vi "_OLS_Main_Rev2.vi"() -> ()   [LabVIEW 2024]
uses:
  Control Definitions/Def Results2.ctl
  Control Definitions/Def PumpCtlRefs.ctl
  Control Definitions/Def_PumpSpeed.ctl
  Control Definitions/Def TestState.ctl
  Control Definitions/Global 1.vi
  Control Definitions/Global 2.vi
panel:
  out "Index Out":i32
  out "TEST State Out":T1
  in  "Pump Speed":T2=enum."SLOW"
  in  "Num Chan":i32=2
  in  "VISA Refnum in":refnum<visa-resource-name>="COM3"
  out "PumpCtlRef out":T3
  in  "SimPV":bool
  out "Ch B  Sim":dbl
  out "Ch A  Sim":dbl
  out "Root Path":path=path "C:/Users/ff107/OneDrive/Documents/GitHub/PWC-OLS"
  out "File Name":string
  out "Time(ms)":dbl=221.000000000016
  in  "Tank Cal Table":T4={"LSe"=8.5, "LKe"=4.0782, "LMe"=5.542, "LKf"=7.004, "LMf"=2.619, "LSf"=2.0}
  out "Level":bool=TRUE
  out "DataQ":bool=TRUE
  in  "ChA":dbl(slide)=24.489795918367346 scale=0.0..1200.0
  in  "ChB":dbl(slide)=36.73469387755102 scale=0.0..1200.0
  in  "ChB +100":bool
  in  "ChA +100":bool
  in  "Check":bool
  out "Laser (raw)":dbl=5.418700218200684
  out "Results out":T5=[[{"Fill"=0.0, "Drain"=0.0, "Status"=1, "Resistor"=100.77651728439153}, {"Fill"=0.0, "Drain"=0.0, "Status"=1, "Resistor"=100.51009270770467}], [{"Fill"=7.4414529208790405, "Drain"=0.0, "Status"=10, "Resistor"=199.9225077433029}, {"Fill"=7.238431105656106, "Drain"=0.0, "Status"=5, "Resistor"=199.90723695805426}], [{"Fill"=7.01332844493592, "Drain"=0.0, "Status"=5, "Resistor"=299.5771992355265}, {"Fill"=6.753456462357763, "Drain"=0.0, "Status"=10, "Resistor"=299.405945542382}], [{"Fill"=6.5453388658426634, "Drain"=0.0, "Status"=10, "Resistor"=398.9472825404134}, {"Fill"=6.2984555038112795, "Drain"=0.0, "Status"=10, "Resistor"=398.8781708461997}], [{"Fill"=6.077648954516121, "Drain"=0.0, "Status"=10, "Resistor"=498.9171881446158}, {"Fill"=5.838658669949018, "Drain"=0.0, "Status"=10, "Resistor"=498.9668209325864}], [{"Fill"=5.635836474430779, "Drain"=0.0, "Status"=10, "Resistor"=599.1164295543886}, {"Fill"=5.372367525813369, "Drain"=0.0, "Status"=10, "Resistor"=599.0753796448585}], [{"Fill"=5.159054576363429, "Drain"=0.0, "Status"=10, "Resistor"=699.4116005363627}, {"Fill"=4.928457133151359, "Drain"=0.0, "Status"=10, "Resistor"=699.1833846499306}], [{"Fill"=4.711946933490899, "Drain"=0.0, "Status"=10, "Resistor"=799.7085090018842}, {"Fill"=4.472056930994641, "Drain"=0.0, "Status"=10, "Resistor"=799.8411539311372}], [{"Fill"=0.0, "Drain"=0.0, "Status"=2, "Resistor"=0.0}, {"Fill"=0.0, "Drain"=0.0, "Status"=0, "Resistor"=0.0}], [{"Fill"=0.0, "Drain"=0.0, "Status"=0, "Resistor"=0.0}, {"Fill"=0.0, "Drain"=0.0, "Status"=0, "Resistor"=0.0}], [{"Fill"=0.0, "Drain"=0.0, "Status"=0, "Resistor"=0.0}, {"Fill"=0.0, "Drain"=0.0, "Status"=0, "Resistor"=0.0}]] {"Resistor" format="%.1f"; "Drain" format="%.3f"; "Fill" format="%.3f"}
  in  "DUT":i16=1
  in  "Pump JOG":bool
  in  "Run Test":bool
  in  "Normal":cluster{u32, u32}[](array[cluster])=[{16711680, 1244948}]
  in  "Sim Color":cluster{u32, u32}[](array[cluster])=[{16774656, 1244948}]
  out "Level \nStatus":bool=TRUE
  out "DataQ\nStatus":bool=TRUE
  in  "Level SP":dbl(slide)=2.6 scale=8.5..2.0
  in  "Level PV":dbl(slide)=4.203692297209104 scale=8.5..2.0
  out "Level":dbl=4.203692297209104 format="%.3f"
  in  "Drain":bool
  in  "Fill":bool
  in  "Simulate":bool
  out "TEST NME":string="OLR001--Junk"
  out "DataQ Input":T6(graph)={"ChA Ohms"=799.7643554010987, "ChB Ohms"=799.7713366200159, "Laser (raw)"=5.343100070953369}
  out "Time Stamp":timestamp=timestamp(3801643928.5713105 s since 1904-01-01)
  in  "stop":bool
  out "ChB Ohms":dbl=799.966848563534 format="%.1f"
  out "ChA Ohms":dbl=899.5202427178965 format="%.1f"
  # "Calibration & Scaling Table\n               Tank         Key          Ref\n               Scale        Level        Measure\n\n\n\nEmpty\n\n\nFull"
  # "8.5   1.7752   7.844\n\n2.0   6.112    3.511"
  # "CHA"
  # "CHB"
  # "Resistance   Fill        Drain"
  # "Resistance   Fill        Drain"
  # "Simulated Instrument Inputs"
  # "PUMP"
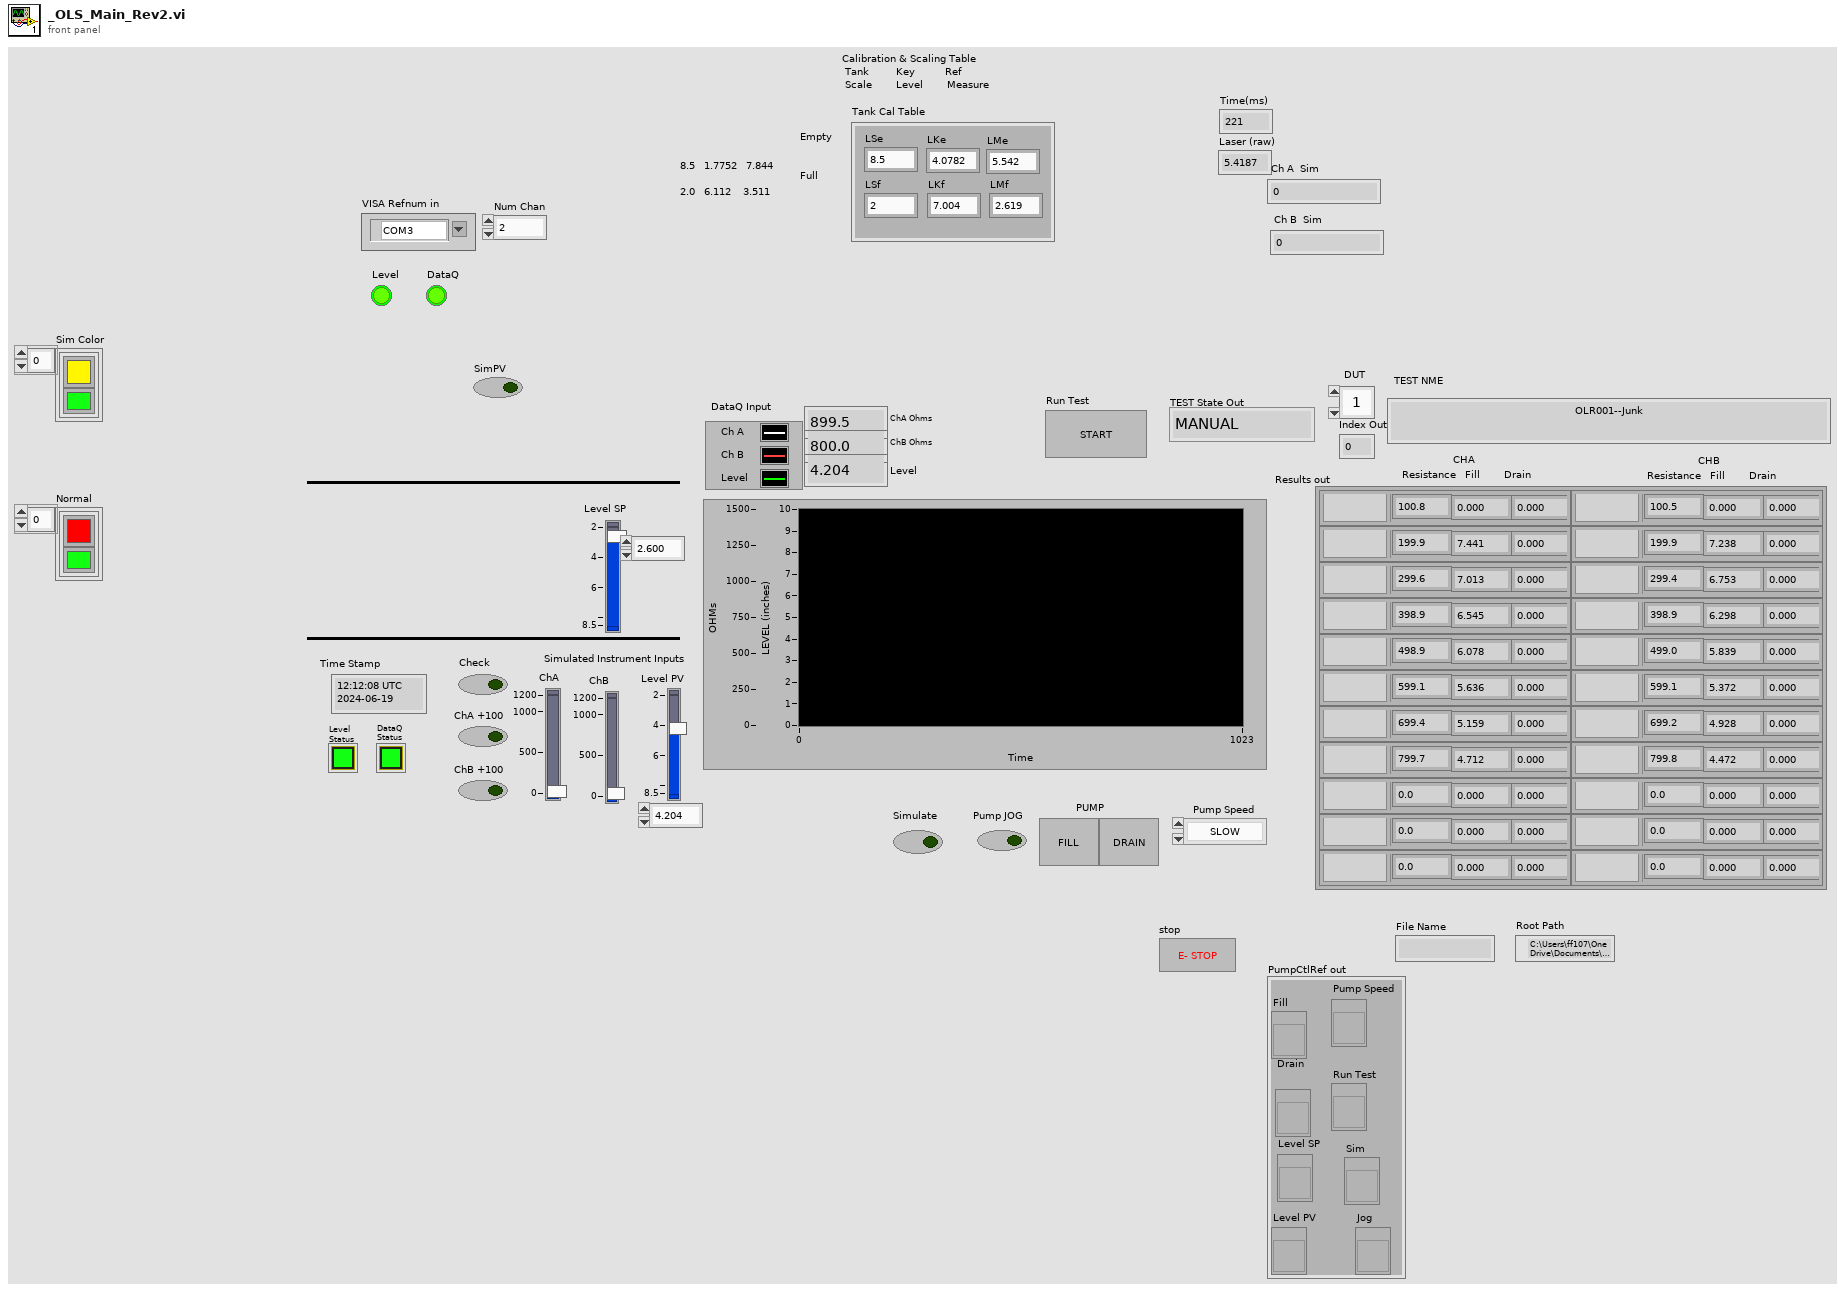
[diagram p1: front panel]
types:
  T1 = typedef "Def TestState.ctl" = enum16{"MANUAL", "Start", "Pre-Fill", "Pre-Drain", "Init-Record", "Load Fill Spec", "Filling Hi", "Wait1", "Record Fill", "Load Drain Spec", "Draining Lo", "Wait2", "Record Drain", "Empty", "Done"}
  T2 = typedef "Def_PumpSpeed.ctl" = enum16{"FAST", "SLOW", "CREEP", "STOP"}
  T3 = typedef "Def PumpCtlRefs.ctl" = cluster{"Fill ":refnum<vi>, "Drain":refnum<vi>, "Level PV":refnum<vi>, "Pump Speed":refnum<vi>, "Run Test":refnum<vi>, "Sim":refnum<vi>, "Jog":refnum<vi>, "Level SP":refnum<vi>}
  T4 = cluster{"LSe":dbl, "LKe":dbl, "LMe":dbl, "LKf":dbl, "LMf":dbl, "LSf":dbl}
  T5 = typedef "Def Results2.ctl" = cluster{"Fill":dbl, "Drain":dbl, "Status":i16, "Resistor":dbl}[][]
  T6 = cluster{"ChA Ohms":dbl, "ChB Ohms":dbl, "Laser (raw)":dbl}
  T7 = cluster{"Level \nStatus":refnum<vi>, "DataQ\nStatus":refnum<vi>}
  T8 = typedef "Def FullCfg.ctl" = cluster{"Bench Config":T9, "Test Value Table ":dbl[][], "Table Col Titles":string[][], "Pump CtlRef In":T3, "Bench Status":T10}
  T9 = typedef "Def BenchCfg.ctl" = cluster{"Name":string, cluster{"Step Levels":dbl, "Tolerance":dbl, "Sample Rate":dbl, "Resistor":dbl, "M Level Cal":dbl, "[B Level Cal":dbl, "Max Fill Rate":dbl, "Empty Inches":dbl, "Full Inches":dbl}}
  T10 = typedef "Def Bench Status.ctl" = cluster{"Pump Status":refnum<vi>, "Instrumnet\n Status":refnum<vi>}
  T11 = typedef "Def CalCoef.ctl" = cluster{"M":dbl, "B":dbl, "Mc":dbl, "Bc":dbl, "LMe":dbl}
  T12 = enum16{"MANUAL", "Start", "Filling", "FULL", "Draining", "EMPTY", "Done"}
  T13 = cluster{"Resistor":dbl, "Fill":dbl, "Drain":dbl, "Status":i16}
  T14 = cluster{"Resistor":dbl, "Fill":dbl, "Drain":dbl, "Status":i16}[][]
  T15 = cluster{"Ch A   Ohms":dbl, " Ch B  Ohms":dbl, "Level OUt":dbl}
  T16 = typedef "DEF_SpecsOut.ctl" = cluster{"aSpecsTable":T17[], "Pump CtlRef In":T3}
  T17 = typedef "Ded Spec RNG.ctl" = cluster{"Specs":dbl[], "Index(n)":i32, "LUT Status":T18, "Index(n-1)":i32}
  T18 = typedef "Ded LUT_Status.ctl" = cluster{"ChA/!ChB":bool, "Drain/!Fill":bool, "In Range?":bool, "Switch Range?":bool, "Measure R?":bool, "Vaild R?":bool}
  T19 = typedef "Def Measure.ctl" = cluster{"ChA R":dbl, "ChB R":dbl, "Level PV":dbl}
  T20 = cluster{"Resistor":dbl, "Fill":dbl, "Drain":dbl, "Resistor":dbl}[][]
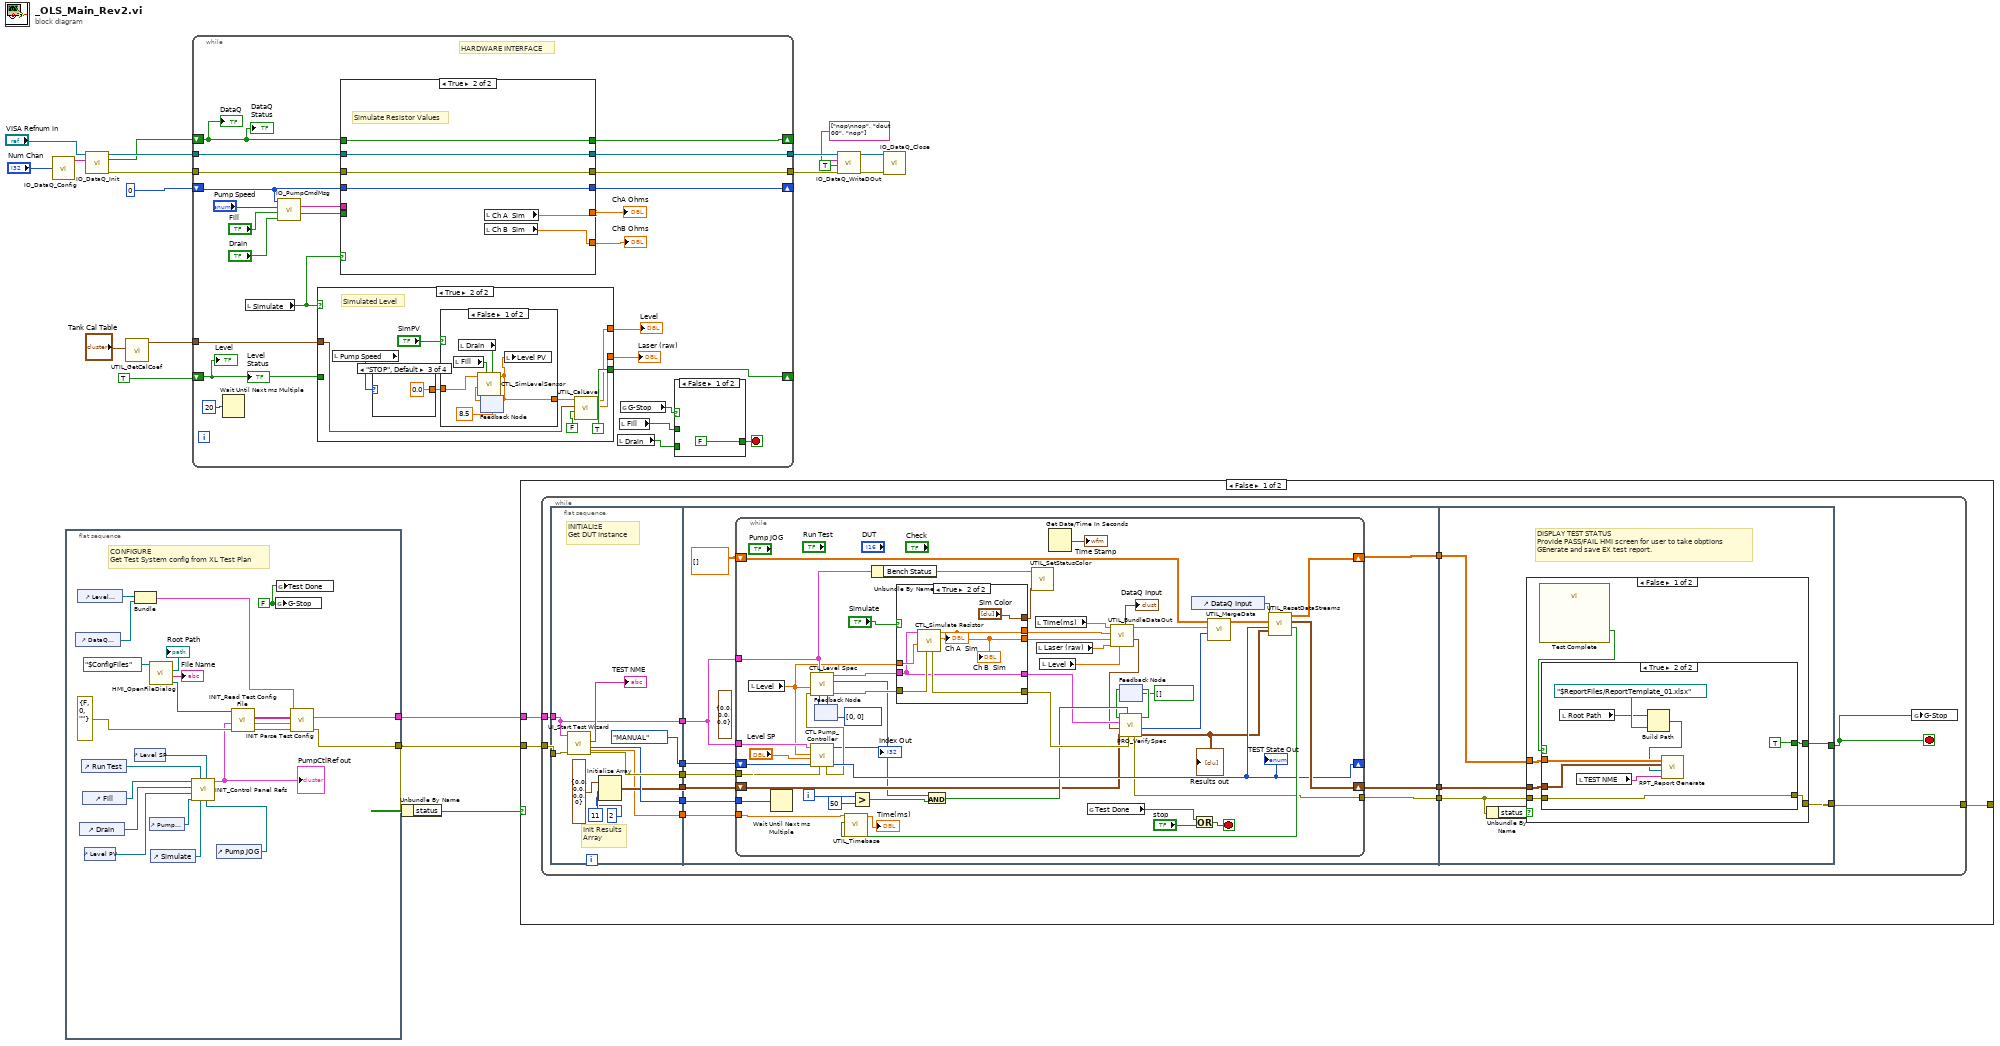
[diagram p0: block diagram]
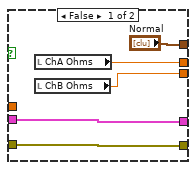
[diagram p2: hidden frame]
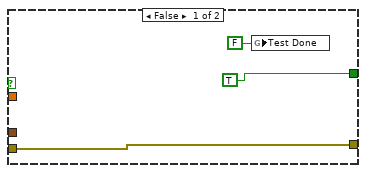
[diagram p3: hidden frame]
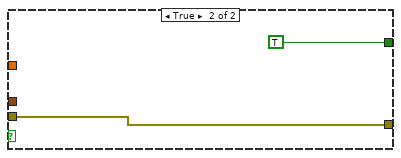
[diagram p4: hidden frame]
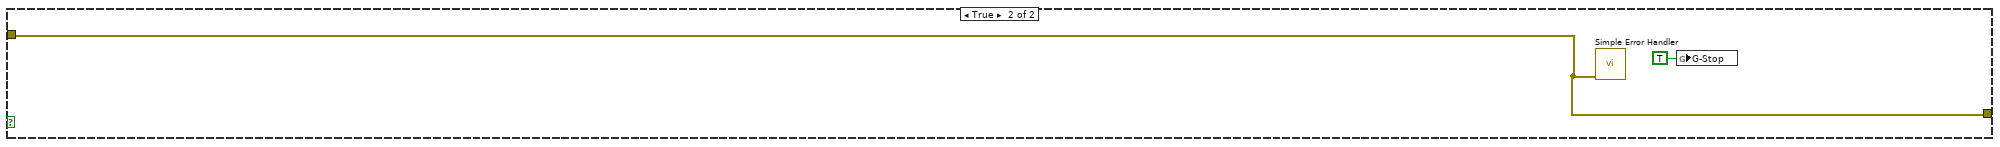
[diagram p5: hidden frame]
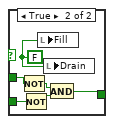
[diagram p6: hidden frame]
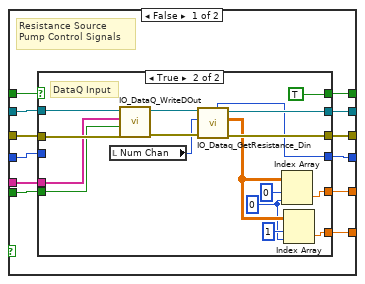
[diagram p7: hidden frame]
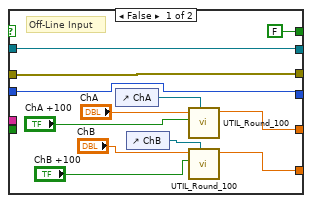
[diagram p8: hidden frame]
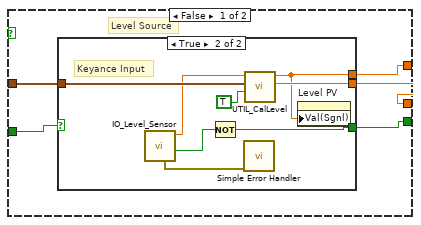
[diagram p9: hidden frame]
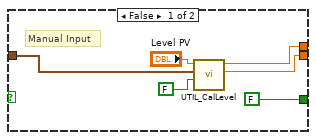
[diagram p10: hidden frame]
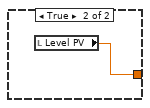
[diagram p11: hidden frame]
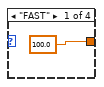
[diagram p12: hidden frame]
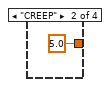
[diagram p13: hidden frame]
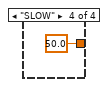
[diagram p14: hidden frame]
diagram:
  n1 = call "IO_DataQ_Config.vi"("Num Chan"="Num Chan") -> ("Init Message"=w19:string[])  [unwired: 10 in]
  n2 = flat-sequence {
    tunnel: [w39] -> w11
    tunnel: [w31] -> w1
    frame #0 {
      w26 = FALSE ("G-Stop")
      # "CONFIGURE\nGet Test System config from XL Test Plan"
      n3 = control-ref of="DataQ\nStatus"() -> (w28:refnum<vi>)
      n4 = control-ref of="Level \nStatus"() -> (w38:refnum<vi>)
      n5 = control-ref of="Drain"() -> (w40:refnum<vi>)
      n6 = control-ref of="Run Test"() -> (w33:refnum<vi>)
      n7 = control-ref of="Fill"() -> (w34:refnum<vi>)
      n8 = control-ref of="Level PV"() -> (w36:refnum<vi>)
      n9 = Bundle("Level \nStatus"=w38, "DataQ\nStatus"=w28) -> (w37:T7)  [unwired: 1 in]
      n10 = control-ref of="Level SP"() -> (w27:refnum<vi>)
      n11 = call "HMI_OpenFileDialog.vi"("relative path"=path "$ConfigFiles") -> ("selected path"=w22:path, "File Name"=→"File Name":string, "Root Path"=→"Root Path":path)  [unwired: 8 in]
      n12 = control-ref of="Pump Speed"() -> (w21:refnum<vi>)
      n13 = control-ref of="Simulate"() -> (w30:refnum<vi>)
      n14 = control-ref of="Pump JOG"() -> (w29:refnum<vi>)
      n15 = call "INIT_Control Panel Refs.vi"("Jog"=w29, "Level SP"=w27, "Sim"=w30, "Run Test"=w33, "Pump Speed"=w21, "Level PV"=w36, "Drain"=w40, "Fill"=w34) -> ("PumpCtlRef out"=w20:T3)  [unwired: 3 in]
      "PumpCtlRef out" <- w20
      n16 = call "INIT_Read Test Config File.vi"("error in (no error)"=errorcluster {"status"=FALSE, "code"=0, "source"=""}, "Path"=w22) -> ("error out 2"=w32:errorcluster, "Config\nFile Data"=w35:string[][])  [unwired: 8 in]
      n17 = global write "Global 1.vi" "G-Stop"(w26) -> ()
      n18 = global write "Global 2.vi" "Test Done"(w26) -> ()
      n19 = call "INIT Parse Test Config.vi"("error in (no error)"=w32, "Pump CtlRef In"=w20, "All XL Input"=w35, "Bench Status"=w37) -> ("error out"=w39:errorcluster, "Full Config"=w31:T8)  [unwired: 6 in]
    }
  }
  n20 = call "IO_DataQ_Init.vi"("Command\nList"=w19, "VISA Refnum in"="VISA Refnum in") -> ("error out"=w17:errorcluster, "Connected?"=w16:bool, "VISA resource name out"=w18:refnum<visa-resource-name>)  [unwired: 7 in]
  n21 = call "UTIL_GetCalCoef.vi"("Cal Table"="Tank Cal Table") -> ("Cal Coef out"=w14:T11)  [unwired: 10 in]
  n22 = while {
    shift-right: [w64] -> _
    shift-left: TRUE ("Pump \nStatus") -> [w44]
    tunnel: w18 -> [w63]
    tunnel: w17 -> [w62]
    tunnel: [w60] -> w10
    tunnel: [w61] -> w8
    shift-right: [w59] -> _
    shift-left: w16 -> [w58]
    tunnel: w14 -> [w56]
    shift-right: [w47] -> _
    shift-left: 0 -> [w43]
    stop <- w53 stop-if-true
    # "HARDWARE INTERFACE"
    n23 = Wait Until Next ms Multiple(millisecond multiple=u32 20) -> ()  [unwired: 1 out]
    n24 = local read "Simulate"() -> (w55:bool)
    n25 = call "IO_PumpCmdMsg.vi"("Drain Signal"="Drain", "FIll Signal"="Fill", "Pump Speed"="Pump Speed", "Cmd IN"=w43) -> ("Msg Active"=w48:bool, "Message"=w57:string[])  [unwired: 4 in, 2 out]
    n26 = case shown="True" w55 {
      tunnel: [w126 w146] -> w42
      tunnel: [w125 w148] -> w65
      tunnel: [w122 TRUE] -> w64
      tunnel: w44 -> [w124 _]
      tunnel: w56 -> [w123 w141]
      frame False {
        # "Level Source"
        n27 = case shown="True" w124 {
          tunnel: [w130 w133] -> w126
          tunnel: [w129 w138] -> w125
          tunnel: [FALSE ("status") w137] -> w122
          tunnel: w123 -> [w131 w139]
          frame False {
            # "Manual Input"
            n28 = call "UTIL_CalLevel.vi"("Key is In?"=FALSE, "Cal Coef in"=w131, "Input"="Level PV") -> ("PVc"=w129:dbl, "PVs"=w130:dbl)  [unwired: 7 in]
          }
          frame True {
            # "Keyance Input"
            n29 = call "IO_Level_Sensor.vi"() -> ("status"=w135:bool, "PV (raw)"=w136:dbl, "error OUT"=w134:errorcluster)  [unwired: 9 in]
            n30 = Not(x=w135) -> (.not. x?=w137:bool)
            n31 = call <vilib>:"Simple Error Handler.vi"("error in (no error)"=w134) -> ()  [unwired: 4 in, 5 out]
            n32 = call "UTIL_CalLevel.vi"("Key is In?"=TRUE, "Cal Coef in"=w139, "Input"=w136) -> ("PVc"=w138:dbl, "PVs"=w133:dbl)  [unwired: 7 in]
            n33 = property on="Level PV" class="Slide (strict)"("Val(Sgnl)"=w133) -> ()  [unwired: 2 in, 2 out]
          }
        }
      }
      frame True {
        # "Simulated Level"
        n34 = local read "Pump Speed"() -> (w144:T2)
        n35 = case shown="\"STOP\", Default" w144 {
          tunnel: [100.0 ("Ctl Sig") 5.0 ("Ctl Sig") 0.0 ("Ctl Sig") 50.0 ("Ctl Sig")] -> w145
          frame "FAST" {
          }
          frame "CREEP" {
          }
          frame "STOP", Default {
          }
          frame "SLOW" {
          }
        }
        n36 = case shown="False" "SimPV" {
          tunnel: w145 -> [w154 _]
          tunnel: [w150 w156] -> w143
          frame False {
            n37 = local read "Fill"() -> (w155:bool)
            n38 = local read "Drain"() -> (w151:bool)
            n39 = feedback #1(8.5 ("PV Level Inch")) -> (w152:dbl)
            n40 = call "CTL_SimLevelSensor.vi"("Drain IN"=w151, "Fill IN"=w155, "Level PV in"=w152, "Pump Speed"=w154) -> ("PV Level Inch"=w150:dbl)  [unwired: 7 in]
            n41 = feedback-in #1(w150) -> ()
            n42 = local write "Level PV"(w150) -> ()
          }
          frame True {
            n43 = local read "Level PV"() -> (w156:dbl)
          }
        }
        n44 = call "UTIL_CalLevel.vi"("Key is In?"=FALSE, "Cal Coef in"=w141, "Input"=w143) -> ("PVc"=w148:dbl, "PVs"=w146:dbl)  [unwired: 7 in]
      }
    }
    "Level" <- w42
    "Laser (raw)" <- w65
    n45 = case shown="True" w55 {
      tunnel: [w86 w118] -> w66
      tunnel: [w85 w117] -> w45
      tunnel: w63 -> [w78 w120]
      tunnel: w62 -> [w80 w119]
      tunnel: [w84 w119] -> w61
      tunnel: [w83 w120] -> w60
      tunnel: [w82 w121] -> w59
      tunnel: w58 -> [w81 w121]
      tunnel: w57 -> [w79 _]
      tunnel: w48 -> [w77 _]
      tunnel: [w76 w116] -> w47
      tunnel: w43 -> [w75 w116]
      frame False {
        # "Resistance Source\nPump Control Signals"
        n46 = case shown="True" w81 {
          tunnel: [w91 w111] -> w86
          tunnel: [w92 w100] -> w85
          tunnel: [w93 w115] -> w83
          tunnel: [w94 w114] -> w84
          tunnel: [FALSE TRUE] -> w82
          tunnel: w80 -> [w94 w109]
          tunnel: w79 -> [_ w105]
          tunnel: w78 -> [w93 w108]
          tunnel: w77 -> [_ w104]
          tunnel: [w87 w101] -> w76
          tunnel: w75 -> [w87 _]
          frame False {
            # "Off-Line Input"
            n47 = control-ref of="ChA"() -> (w90:refnum<vi>)
            n48 = control-ref of="ChB"() -> (w88:refnum<vi>)
            n49 = call "UTIL_Round_100.vi"("Num Refnum"=w90, "100"="ChA +100", "IN"="ChA") -> ("OUT"=w92:dbl)  [unwired: 8 in]
            n50 = call "UTIL_Round_100.vi"("Num Refnum"=w88, "100"="ChB +100", "IN"="ChB") -> ("OUT"=w91:dbl)  [unwired: 8 in]
          }
          frame True {
            w99 = 0 ("disabled index (col)")
            # "DataQ Input"
            n51 = local read "Num Chan"() -> (w102:i32)
            n52 = call "IO_DataQ_WriteDOut.vi"("error in (no error)"=w109, "Msg Active"=w104, "Message"=w105, "VISA Refnum in"=w108) -> ("error out"=w107:errorcluster, "VISA Refnum out"=w106:refnum<visa-resource-name>)  [unwired: 6 in]
            n53 = call "IO_Dataq_GetResistance_Din.vi"("error in (no error)"=w107, "Num Chan"=w102, "VISA Refnum in"=w106) -> ("error out"=w114:errorcluster, "Analog"=w103:dbl[][], "VISA Refnum out"=w115:refnum<visa-resource-name>, "Cmd"=w101:u32)  [unwired: 3 in, 2 out]
            n54 = Index Array(array=w103, index (row)=0 ("index"), index (col)=w99) -> (element=w100:dbl)
            n55 = Index Array(array=w103, index (row)=1 ("index"), index (col)=w99) -> (element=w111:dbl)
          }
        }
      }
      frame True {
        # "Simulate Resistor Values"
        n56 = local read "Ch A  Sim"() -> (w117:dbl)
        n57 = local read "Ch B  Sim"() -> (w118:dbl)
      }
    }
    "ChA Ohms" <- w45
    "ChB Ohms" <- w66
    n58 = local read "Drain"() -> (w51:bool)
    n59 = local read "Fill"() -> (w52:bool)
    n60 = global read "Global 1.vi" "G-Stop"() -> (w54:bool)
    n61 = case shown="False" w54 {
      tunnel: [FALSE w70] -> w53
      tunnel: w52 -> [_ w72]
      tunnel: w51 -> [_ w69]
      frame False {
      }
      frame True {
        w74 = FALSE
        n62 = Not(x=w72) -> (.not. x?=w73:bool)
        n63 = Not(x=w69) -> (.not. x?=w71:bool)
        n64 = local write "Fill"(w74) -> ()
        n65 = local write "Drain"(w74) -> ()
        n66 = And(x=w73, y=w71) -> (x .and. y?=w70:bool)
      }
    }
    "DataQ\nStatus" <- w58
    "Level \nStatus" <- w44
    "DataQ" <- w58
    "Level" <- w44
  }
  n67 = Unbundle By Name(w11) -> ("status"=w13:bool)
  n68 = case shown="False" w13 {
    tunnel: w11 -> [w163 w287]
    tunnel: w1 -> [w162 _]
    tunnel: [w161 w287] -> _
    frame False {
      n69 = while {
        tunnel: w163 -> [w173]
        tunnel: w162 -> [w171]
        tunnel: [w166] -> w161
        stop <- w165 stop-if-true
        n70 = flat-sequence {
          tunnel: [w185] -> w175
          tunnel: [w186] -> w174
          tunnel: w173 -> [w187]
          tunnel: [w177] -> w172
          tunnel: w171 -> [w177]
          tunnel: [T12."MANUAL" ("TEST STATUS Out")] -> w170
          tunnel: [w180] -> w169
          tunnel: [w179] -> w164
          tunnel: [w191] -> w176
          tunnel: w175 -> [w196]
          tunnel: w174 -> [w197]
          tunnel: w172 -> [w188]
          tunnel: w170 -> [w189]
          tunnel: w169 -> [w195]
          tunnel: [w194] -> w168
          tunnel: [w193] -> w167
          tunnel: w164 -> [w192]
          tunnel: w176 -> [w267]
          tunnel: [w266] -> w165
          tunnel: [w264] -> w166
          tunnel: w168 -> [w263]
          tunnel: w167 -> [w262]
          frame #0 {
            # "Init Results\nArray"
            # "INITIALIzE\nGet DUT Instance"
            n71 = call "UI_Start Test Wizard.vi"("error in (no error)"=w187, "Full Config"=w177) -> ("error out"=w186:errorcluster, "Time Base mS"=w185:i32, "Title"=→"TEST NME":string, "Sample Rate"=w179:dbl)  [unwired: 4 in]
            n72 = Initialize Array(T13 {"Resistor"=0.0, "Fill"=0.0, "Drain"=0.0, "Status"=0} ("Cluster 2"), 11 ("dimension size"), 2 ("dimension size")) -> (w180:T14)
          }
          frame #1 {
            (unwired) T15 {"Ch A   Ohms"=0.0, " Ch B  Ohms"=0.0, "Level OUt"=0.0}
            n73 = while {
              tunnel: w196 -> [w247]
              tunnel: w197 -> [w235]
              tunnel: [w222] -> w191
              tunnel: w188 -> [w200]
              shift-right: [w229] -> w193
              shift-left: w195 -> [w221]
              tunnel: w192 -> [w234]
              shift-right: [w230] -> w194
              shift-left: dbl[][] [] ("Array") -> [w212]
              shift-right: [w226] -> _
              shift-left: w189 -> [w225]
              tunnel: w188 -> [w207]
              i -> [w233]
              stop <- w244 stop-if-true
              n74 = local read "Level"() -> (w199:dbl)
              n75 = Wait Until Next ms Multiple(millisecond multiple=w247) -> ()  [unwired: 1 out]
              n76 = call "CTL Pump_Controller.vi"("error in (no error)"=w235, "TEST State In"=w225, "Level SP"="Level SP", "Level PV"=w199, "Full Cfg"=w207) -> ("TEST State Out"=w226:T1, "Index Out"=→"Index Out":i32, "error out"=w206:errorcluster)  [unwired: 1 in, 3 out]
              "TEST State Out" <- w226
              n77 = feedback #2(i32[] [0, 0] ("Index(n-1) In")) -> (w203:i32[])
              n78 = call "CTL_Level Spec.vi"("Index(n-1) In"=w203, "Full Config 2"=w200, "error in (no error)"=w206, "Level IN inches"=w199) -> ("error out"=w205:errorcluster, "Enable"=w201:bool, "Specs Out"=w202:T16, "Index(n-1) Out"=w204:i32[])  [unwired: 4 in]
              n79 = feedback-in #2(w204) -> ()
              n80 = Greater?(x=w233, y=50) -> (0:w231:bool)
              n81 = Unbundle By Name(w200) -> ("Bench Status"=w245:T10)
              n82 = case shown="True" "Simulate" {
                tunnel: w205 -> [w254 w257]
                tunnel: [w254 w260] -> w224
                tunnel: ["Normal" "Sim Color"] -> w246
                tunnel: [w252 w259] -> w238
                tunnel: [w251 w258] -> w237
                tunnel: w202 -> [w250 w255]
                tunnel: w199 -> [_ w256]
                tunnel: [w250 w255] -> w220
                frame False {
                  n83 = local read "ChA Ohms"() -> (w252:dbl)
                  n84 = local read "ChB Ohms"() -> (w251:dbl)
                }
                frame True {
                  n85 = call "CTL_Simulate Resistor.vi"("error in (no error)"=w257, "Level IN"=w256, "Specs IN"=w255) -> ("Ch B  Ohms"=w258:dbl, "Ch A  Ohms"=w259:dbl, "error out"=w260:errorcluster)  [unwired: 6 in]
                  "Ch A  Sim" <- w259
                  "Ch B  Sim" <- w258
                }
              }
              n86 = And(x=w201, y=w231) -> (x .and. y?=w223:bool)
              n87 = call "UTIL_SetStatusColor.vi"("Colors [4] in"=w246, "Bench Status"=w245) -> ()  [unwired: 10 in]
              n88 = local read "Time(ms)"() -> (w241:dbl)
              n89 = local read "Laser (raw)"() -> (w240:dbl)
              n90 = local read "Level"() -> (w208:dbl)
              n91 = Get Date/Time In Seconds() -> (seconds since 1Jan1904=→"Time Stamp":timestamp)
              n92 = global read "Global 2.vi" "Test Done"() -> (w242:bool)
              n93 = call "UTIL_BundleDataOut.vi"("Level PV"=w208, "Laser (raw)"=w240, "ChB Ohms"=w237, "ChA Ohms"=w238, "Time (ms)"=w241) -> ("Measure"=w219:T19, "Data Out"=w214:dbl[], "Chart Data"=→"DataQ Input":T6)  [unwired: 3 in, 1 out]
              n94 = feedback #3(bool[] [] ("Switched Out")) -> (w216:bool[])
              n95 = call "PRO_VerifySpec.vi"("error in (no error)"=w224, "Enable"=w223, "Results in"=w221, "Measure In"=w219, "Specs In"=w220, "Switched In"=w216) -> ("Results out"=w218:T5, "Status Code"=w213:i32, "Switched Out"=w217:bool[], "error out"=w222:errorcluster)  [unwired: 2 in]
              "Results out" <- w218
              n96 = feedback-in #3(w217) -> ()
              n97 = control-ref of="DataQ Input"() -> (w209:refnum<vi>)
              n98 = Or(x=w242, y="stop") -> (x .or. y?=w244:bool)
              n99 = call "UTIL_MergeData.vi"("Status Code"=w213, "New Data"=w214, "Data In"=w212) -> ("Data out"=w211:dbl[][])  [unwired: 8 in]
              n100 = call "UTIL_ResetDataStreams.vi"("Results in"=w218, "TEST State Out"=w226, "Data in"=w211, "WaveformChart in"=w209) -> ("Value (Signaling)"=w227:bool, "Results out 2"=w229:T20, "Array"=w230:dbl[][])  [unwired: 5 in]
              n101 = call "UTIL_Timebase.vi"("Reset"=w227, "Sample Rate"=w234) -> ("Time(ms)"=→"Time(ms)":dbl)  [unwired: 9 in]
            }
          }
          frame #2 {
            # "DISPLAY TEST STATUS\nProvide PASS/FAIL HMI screen for user to take obptions\nGEnerate and save EX test report."
            n102 = Unbundle By Name(w267) -> ("status"=w265:bool)
            n103 = case shown="False" w265 {
              tunnel: w267 -> [w271 w285]
              tunnel: [w272 TRUE] -> w266
              tunnel: [w270 w285] -> w264
              tunnel: w263 -> [w269 _]
              tunnel: w262 -> [w268 _]
              frame False {
                n104 = call "Test Complete"() -> ("SAVE"=w273:bool)  [unwired: 18 in, 1 out]
                n105 = case shown="True" w273 {
                  tunnel: [TRUE TRUE] -> w272
                  tunnel: w271 -> [w275 w283]
                  tunnel: [w275 w283] -> w270
                  tunnel: w269 -> [_ w282]
                  tunnel: w268 -> [_ w281]
                  frame False {
                    n106 = global write "Global 2.vi" "Test Done"(FALSE ("Test Done")) -> ()
                  }
                  frame True {
                    n107 = local read "Root Path"() -> (w279:path)
                    n108 = local read "TEST NME"() -> (w277:string)
                    n109 = Build Path(base path=w279, name or relative path=path "$ReportFiles/ReportTemplate_01.xlsx") -> (appended path=w278:path)
                    n110 = call "RPT_Report Generate.vi"("Report Name"=w277, "template"=w278, "Results"=w281, "Wave Data"=w282) -> ()  [unwired: 8 in]
                  }
                }
              }
              frame True {
              }
            }
          }
        }
        n111 = global write "Global 1.vi" "G-Stop"(w165) -> ()
      }
    }
    frame True {
      n112 = call <vilib>:"Simple Error Handler.vi"("error in (no error)"=w287) -> ()  [unwired: 4 in, 5 out]
      n113 = global write "Global 1.vi" "G-Stop"(TRUE ("G-Stop")) -> ()
    }
  }
  n114 = call "IO_DataQ_WriteDOut.vi"("error in (no error)"=w8, "Msg Active"=TRUE, "Message"=string[] ["nop\nnop", "dout 00", "nop"], "VISA Refnum in"=w10) -> ("error out"=w7:errorcluster, "VISA Refnum out"=w9:refnum<visa-resource-name>)  [unwired: 6 in]
  n115 = call "IO_DataQ_Close.vi"("error in"=w7, "VISA resource name"=w9) -> ()  [unwired: 9 in, 1 out]
